vi "Write return.vi"(8 "error in (no error)":errorcluster, 10 "return":i32, 11 "StellarNetSpecAcquisition in":refnum<class "StellarNetSpecAcquisition.lvclass">) -> (0 "error out":errorcluster, 3 "StellarNetSpecAcquisition out":refnum<class "StellarNetSpecAcquisition.lvclass">)   [LabVIEW 2013, in "StellarNetSpecAcquisition.lvclass"]
uses:
  StellarNetSpecAcquisition.lvclass
  StellarNetSpecAcquisition.lvclass/StellarNetSpecAcquisition.ctl
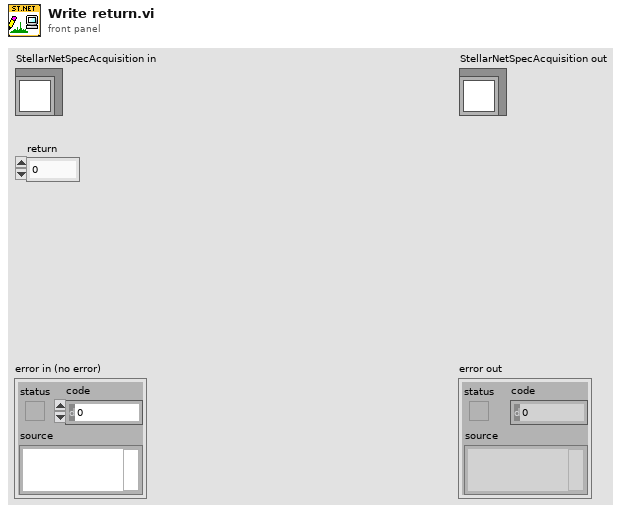
[diagram p1: front panel]
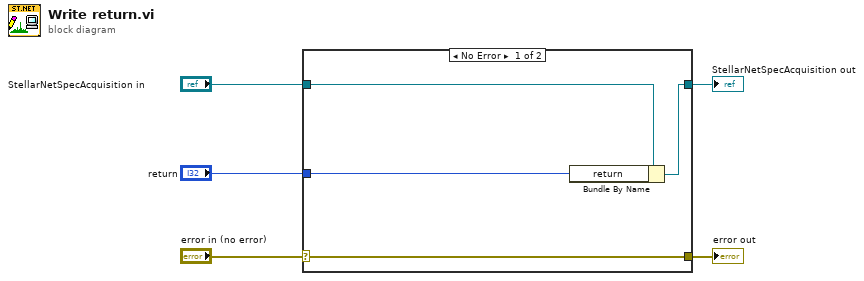
[diagram p0: block diagram]
diagram:
  n1 = case shown="No Error" "error in (no error)" {
    selector: "error in (no error)" -> [w9 w10]
    tunnel: [w9 w10] -> w4
    tunnel: [w7 w11] -> w2
    tunnel: "StellarNetSpecAcquisition in" -> [w8 w11]
    tunnel: "return" -> [w6 _]
    frame No Error {
      n2 = Bundle By Name(cluster=w8, "return"=w6) -> (w7:refnum<class "StellarNetSpecAcquisition.lvclass">)
    }
    frame Error {
    }
  }
  "error out" <- w4
  "StellarNetSpecAcquisition out" <- w2
